vi "Init.vi"(8 "error in (no error)":errorcluster) -> (0 "error out":errorcluster)   [LabVIEW 2017]
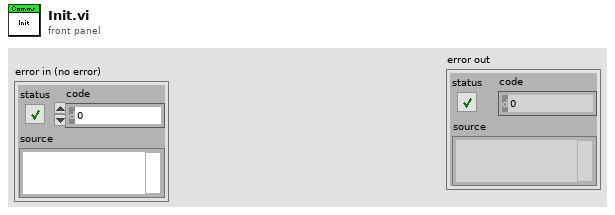
[diagram p1: front panel]
types:
  T1 = enum16{"Init", "Get Index", "Analyze Part", "Analyze Prts", "Analyze Prta", "Set VER", "Set TYPE"}
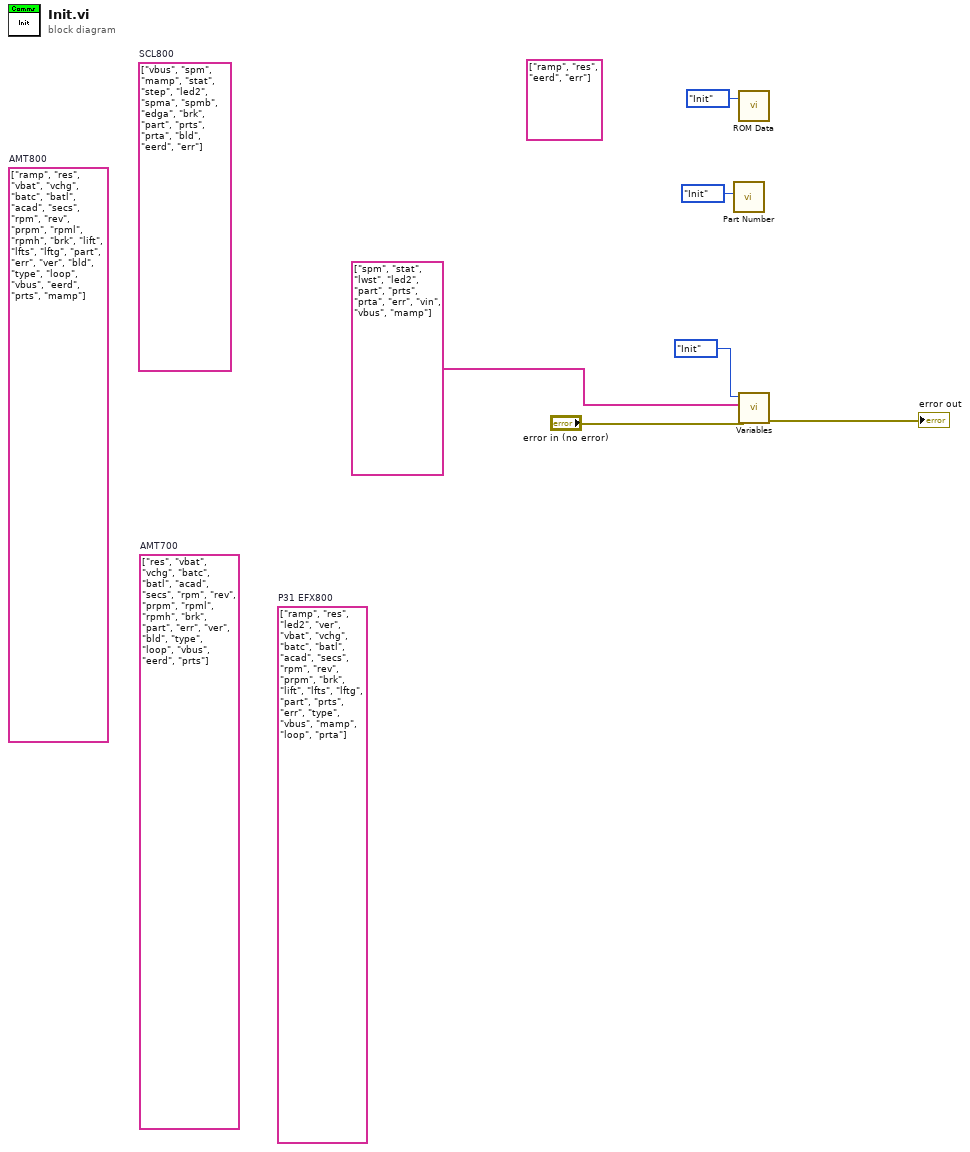
[diagram p0: block diagram]
diagram:
  (unwired) string[] ["vbus", "spm", "mamp", "stat", "step", "led2", "spma", "spmb", "edga", "brk", "part", "prts", "prta", "bld", "eerd", "err"]  # SCL800
  (unwired) string[] ["res", "vbat", "vchg", "batc", "batl", "acad", "secs", "rpm", "rev", "prpm", "rpml", "rpmh", "brk", "part", "err", "ver", "bld", "type", "loop", "vbus", "eerd", "prts"]  # AMT700
  (unwired) string[] ["ramp", "res", "led2", "ver", "vbat", "vchg", "batc", "batl", "acad", "secs", "rpm", "rev", "prpm", "brk", "lift", "lfts", "lftg", "part", "prts", "err", "type", "vbus", "mamp", "loop", "prta"]  # P31 EFX800
  (unwired) string[] ["ramp", "res", "eerd", "err"]
  (unwired) string[] ["ramp", "res", "vbat", "vchg", "batc", "batl", "acad", "secs", "rpm", "rev", "prpm", "rpml", "rpmh", "brk", "lift", "lfts", "lftg", "part", "err", "ver", "bld", "type", "loop", "vbus", "eerd", "prts", "mamp"]  # AMT800
  n1 = call "Part Number.vi"("Command"=T1."Init") -> ()  [unwired: 5 in, 6 out]
  n2 = call "ROM Data.vi"("Command"=enum16{"Init", "Get Index", "Analyze"}."Init") -> ()  [unwired: 1 in, 2 out]
  n3 = call "Variables.vi"("error in (no error)"="error in (no error)", "Value"=string[] ["spm", "stat", "lwst", "led2", "part", "prts", "prta", "err", "vin", "vbus", "mamp"], "Command"=enum16{"Init", "Get", "Set Step Counter"}."Init") -> ("error out"=→"error out":errorcluster)  [unwired: 6 in, 2 out]
